vi "Set Container.vi"(7 "Container":T1, 8 "error in (no error)":errorcluster, 10 "Open/Close (Close)":bool, 11 "cRIO-CO2 in":refnum<class "cRIO-CO2.lvclass">) -> (0 "error out":errorcluster, 3 "cRIO-CO2 out":refnum<class "cRIO-CO2.lvclass">)   [LabVIEW 2015, in "cRIO-Carbondioxide.lvlib" / "cRIO-CO2.lvlib" / "cRIO-CO2.lvclass"]
uses:
  cRIO-CO2.lvclass
  Controls/Sample Transfer Container Enumerator.ctl
  cRIO-CO2.lvclass/cRIO-CO2.ctl
  Sample Line Messages/Open Line Msg/Open Line Msg.lvclass/Open Line Msg.ctl
  <vilib>/ActorFramework/Message Enqueuer/Message Enqueuer.lvclass/Message Enqueuer.ctl
  Storage Line/Storage Line.lvclass
  CO2 Actor Messages/Ping Msg/Ping Msg.lvclass/Ping Msg.ctl
  Storage Line/Storage Line.lvclass/Storage Line.ctl
  Storage Line Messages/Set Line Msg/Set Line Msg.lvclass/Set Line Msg.ctl
  <vilib>/ActorFramework/Message Enqueuer/Enqueue.vi
  <vilib>/ActorFramework/Message Priority Queue/Priority Enqueue.vi
  Interlocks/Interlock Chain/Interlock Chain.lvclass
  Sample Line Messages/Open Line Msg/Open Line Msg.lvclass
  CO2 Actor Messages/Ping Msg/Ping Msg.lvclass
  <vilib>/ActorFramework/Actor/Actor.lvclass
  Storage Line Messages/Set Line Msg/Set Line Msg.lvclass
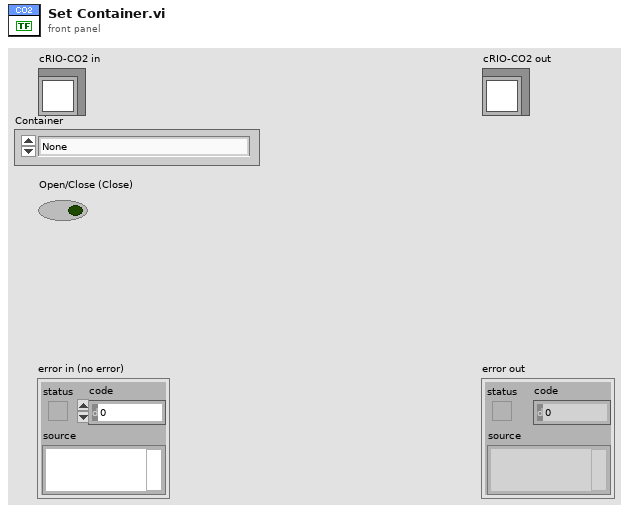
[diagram p1: front panel]
types:
  T1 = typedef "Sample Transfer Container Enumerator.ctl" = enum16{"None", "Sample 1", "Sample 2", "Sample 3", "Sample 4", "Sample 5", "Storage 01", "Storage 02", "Storage 03", "Storage 04", "Storage 05", "Storage 06", "Storage 07", "Storage 08", "Storage 09", "Storage 10", "Storage 11", "Storage 12", "Syringe", "Undefined"}
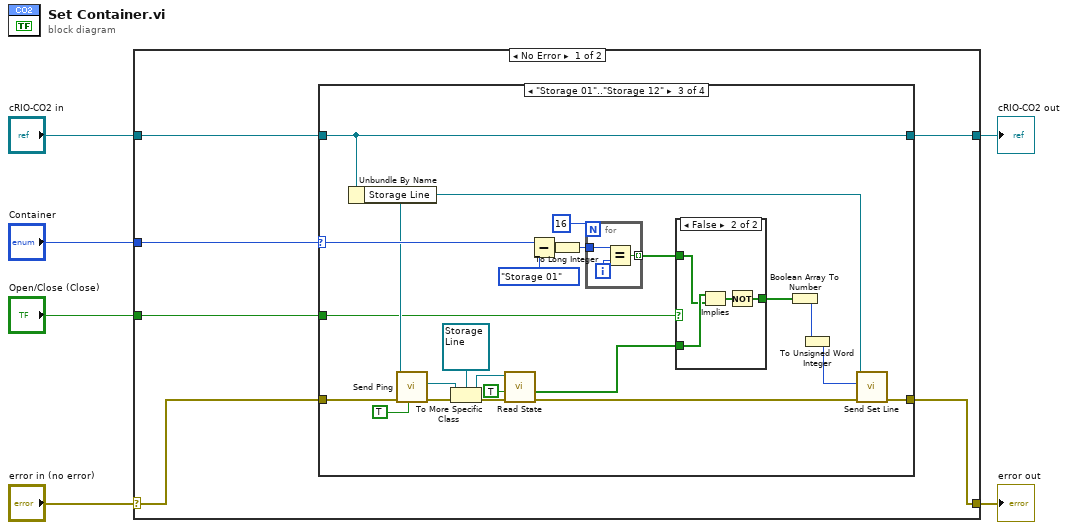
[diagram p0: block diagram]
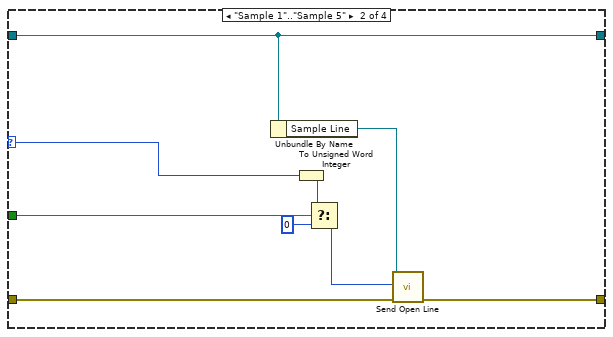
[diagram p3: hidden frame]
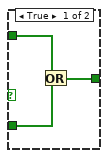
[diagram p4: hidden frame]
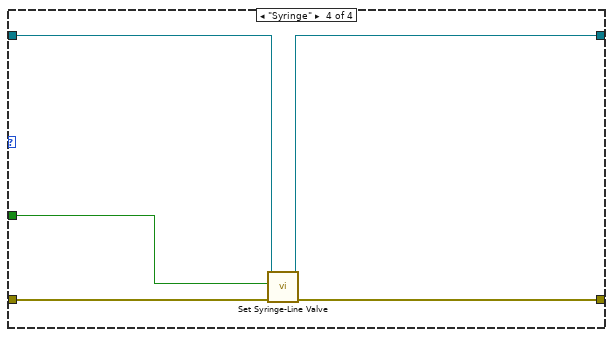
[diagram p5: hidden frame]
diagram:
  n1 = case shown="No Error" "error in (no error)" {
    selector: "error in (no error)" -> [w9 w63]
    tunnel: [w12 w63] -> w5
    tunnel: [w11 w62] -> w3
    tunnel: "cRIO-CO2 in" -> [w10 w62]
    tunnel: "Open/Close (Close)" -> [w8 _]
    tunnel: "Container" -> [w7 _]
    frame No Error {
      n2 = case shown="\"Storage 01\"..\"Storage 12\"" w7 {
        selector: w7 -> [_ w21 w44 _]
        tunnel: w9 -> [w13 w22 w39 w61]
        tunnel: w10 -> [w14 w20 w46 w60]
        tunnel: [w14 w20 w46 w59] -> w11
        tunnel: [w13 w19 w45 w58] -> w12
        tunnel: w8 -> [_ w15 w30 w57]
        frame "Undefined", Default {
        }
        frame "Sample 1".."Sample 5" {
          n3 = Unbundle By Name(w20) -> ("Sample Line"=w23:refnum<class "Message Enqueuer.lvclass">)
          n4 = To Unsigned Word Integer(number=w21) -> (unsigned 16bit integer=w18:u16)
          n5 = Select(t=w18, s=w15, f=u16 0) -> (s? t:f=w17:u16)
          n6 = call "Send Open Line.vi"("error in (no error)"=w22, "Sample Line (All Closed)"=w17, "Message Enqueuer"=w23) -> ("error out"=w19:errorcluster)  [unwired: 7 in, 1 out]
        }
        frame "Storage 01".."Storage 12" {
          n7 = Unbundle By Name(w46) -> ("Storage Line"=w38:refnum<class "Message Enqueuer.lvclass">)
          n8 = call "Send Ping.vi"("Return Self (F)"=TRUE, "error in (no error)"=w39, "Message Enqueuer"=w38) -> ("error out"=w36:errorcluster, "Actor out"=w34:refnum<class "Actor.lvclass">)  [unwired: 5 in, 2 out]
          n9 = To More Specific Class(target class=refnum<class "Storage Line.lvclass"> refnum ("Storage Line.lvclass"), reference=w34, error in=w36) -> (specific class reference=w31:refnum<class "Storage Line.lvclass">, error out=w33:errorcluster)
          n10 = call "Read State.vi"("error in (no error)"=w33, "Return Boolean Array? (F)"=TRUE, "Storage Line in"=w31) -> ("error out"=w32:errorcluster, "Boolean array"=w28:bool[])  [unwired: 4 in, 3 out]
          n11 = Subtract(x=w44, y=Sample_Transfer_Container_Enumerator."Storage 01") -> (x-y=w40:u16)
          n12 = To Long Integer(number=w40) -> (32bit integer=w41:i32)
          n13 = for {
            N: 16 -> [_]
            tunnel: w41 -> [w56]
            tunnel: [w54] -> w27 mode=indexing
            i -> [w55]
            n14 = Equal?(x=w56, y=w55) -> (x = y?=w54:bool)
          }
          n15 = case shown="False" w30 {
            tunnel: w28 -> [w48 w53]
            tunnel: w27 -> [w49 w50]
            tunnel: [w47 w51] -> w26
            frame True {
              n16 = Or(x=w49, y=w48) -> (x .or. y?=w47:bool[])
            }
            frame False {
              n17 = Implies(1:w50, 2:w53) -> (0:w52:bool[])
              n18 = Not(x=w52) -> (.not. x?=w51:bool[])
            }
          }
          n19 = Boolean Array To Number(Boolean array=w26) -> (number=w25:u32)
          n20 = To Unsigned Word Integer(number=w25) -> (unsigned 16bit integer=w24:u16)
          n21 = call "Send Set Line.vi"("error in (no error)"=w32, "Bit Field"=w24, "Message Enqueuer"=w38) -> ("error out"=w45:errorcluster)  [unwired: 7 in, 1 out]
        }
        frame "Syringe" {
          n22 = call "Set Syringe-Line Valve.vi"("error in (no error)"=w61, "ON/OFF(OFF)"=w57, "cRIO-CO2 in"=w60) -> ("error out"=w58:errorcluster, "cRIO-CO2 out"=w59:refnum<class "cRIO-CO2.lvclass">)  [unwired: 7 in]
        }
      }
    }
    frame Error {
    }
  }
  "error out" <- w5
  "cRIO-CO2 out" <- w3
